vi "Get_Time.vi"(0 "error in":errorcluster) -> (1 "error in 2":errorcluster, 2 "seconds since 1Jan1904":timestamp)   [LabVIEW 2010]
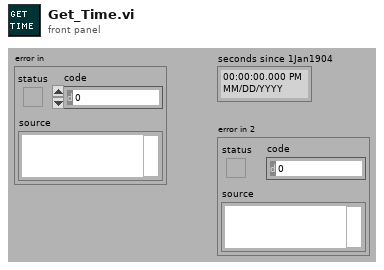
[diagram p1: front panel]
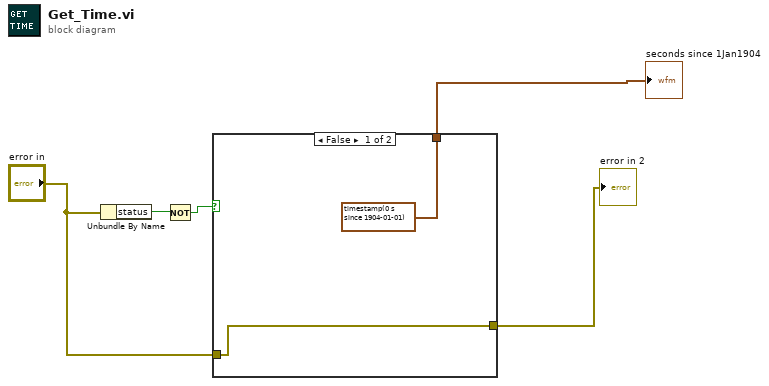
[diagram p0: block diagram]
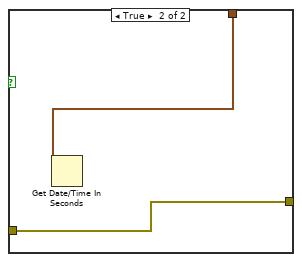
[diagram p2: hidden frame]
diagram:
  n1 = Unbundle By Name("error in") -> ("status"=w5:bool)
  n2 = Not(x=w5) -> (.not. x?=w4:bool)
  n3 = case shown="False" w4 {
    tunnel: [w7 w9] -> w2
    tunnel: "error in" -> [w7 w9]
    tunnel: [timestamp(0 s since 1904-01-01) w8] -> w1
    frame False {
    }
    frame True {
      n4 = Get Date/Time In Seconds() -> (seconds since 1Jan1904=w8:timestamp)
    }
  }
  "seconds since 1Jan1904" <- w1
  "error in 2" <- w2
